vi "Get General Setup.vi"(8 "error in (no error)":errorcluster, 11 "Map":T1) -> (0 "error out":errorcluster, 1 "General Setup":T2={"Export Path"=path "C:/123", "level"=0.8, "Time Gap"=20.0}, 3 "Map Out":T1)   [LabVIEW 2015, in "ConfigHelper.lvlib"]
uses:
  ConfigHelper.lvlib
  Control_General Setup (Path).ctl
  <vilib>/addons/PointValueMap/controls/PointMap.ctl
  <vilib>/addons/PointValueMap/subVIs/Point_Read_variant.vi
  <vilib>/addons/PointValueMap/PointValueMap.lvlib
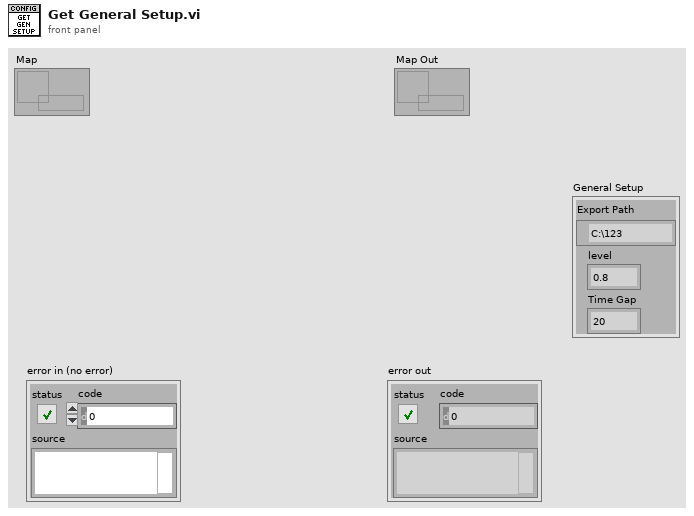
[diagram p1: front panel]
types:
  T1 = typedef "PointValueMap.lvlib/PointMap.ctl" = refnum<data-value>
  T2 = typedef "ConfigHelper.lvlib/Control_General Setup (Path).ctl" = cluster{"Export Path":path, "level":dbl, "Time Gap":dbl}
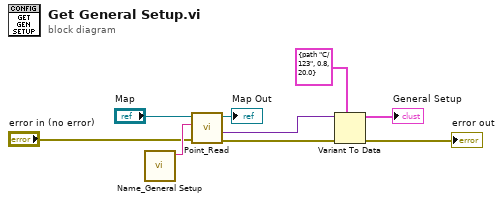
[diagram p0: block diagram]
diagram:
  n1 = call "Name_General Setup.vi"() -> ("Name"=w9:string)  [unwired: 11 in]
  n2 = call-poly <vilib>:"Point_Read.vi"("Error In"="error in (no error)", "Tag"=w9, "Map"="Map") -> ("Error Out"=w8:errorcluster, "Value"=w7:variant, "Map Out"=→"Map Out":T1)  [unwired: 3 in, 3 out]
  n3 = Variant To Data(error in=w8, type=T2 {"Export Path"=path "C:/123", "level"=0.8, "Time Gap"=20.0} ("General Setup"), Variant=w7) -> (data=→"General Setup":T2, error out=→"error out":errorcluster)
